vi "Stop Core.vi"(10 "final error code":i32, 11 "Actor in":refnum<class "Actor.lvclass">) -> (3 "Actor out":refnum<class "Actor.lvclass">)   [LabVIEW 2017, in "Actor Framework.lvlib" / "Actor.lvclass"]
doc: "(<B>Filename</B>: Actor Framework.lvlib:Actor.lvclass:Stop Core.vi)\n\nDefines what the actor does before it stops. Use the <B>final error code</B> input to determine whether the actor shut down in response to an error.\n\nBy default, this method does nothing. A descendant class may override it to define behavior, such as shutting down any processes the actor initiated in its override of the Actor Core method."
uses:
  <vilib>/ActorFramework/Actor/Actor.lvclass
  <vilib>/ActorFramework/Actor/Actor.lvclass/Actor.ctl
  <vilib>/ActorFramework/Message Enqueuer/Message Enqueuer.lvclass
  <vilib>/ActorFramework/Stop Msg/Stop Msg.lvclass/Stop Msg.ctl
  <vilib>/ActorFramework/Message Enqueuer/Message Enqueuer.lvclass/Message Enqueuer.ctl
  <vilib>/ActorFramework/Stop Msg/Send Emergency Stop.vi
  <vilib>/ActorFramework/Stop Msg/Send Normal Stop.vi
  <vilib>/ActorFramework/Message Enqueuer/Enqueue Critical.vi
  <vilib>/ActorFramework/Message Enqueuer/Enqueue.vi
  <vilib>/ActorFramework/Stop Msg/Stop Msg.lvclass
  e:/builds/penguin/labview/branches/2017/dev/dist/vi.lib/ActorFramework/Message/Message.lvclass
  <vilib>/ActorFramework/Message Priority Queue/Priority Enqueue.vi
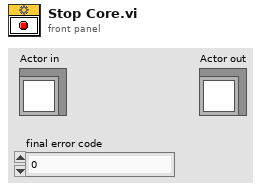
[diagram p1: front panel]
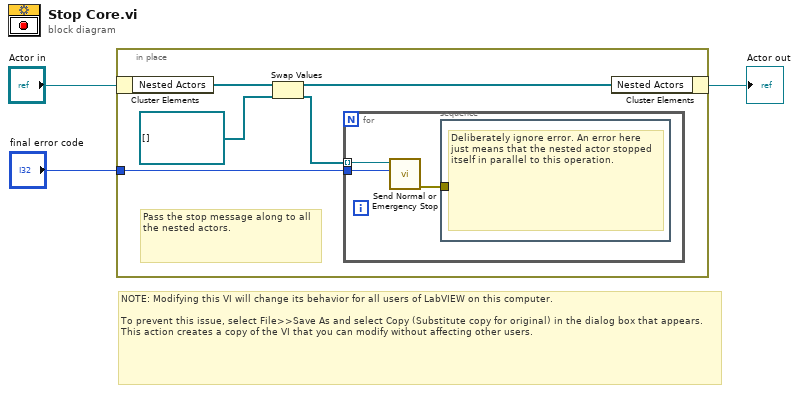
[diagram p0: block diagram]
diagram:
  # "NOTE: Modifying this VI will change its behavior for all users of LabVIEW on this computer.\n\nTo prevent this issue, select File>>Save As and select Copy (Substitute copy for original) in the dialog box that appears. This action creates a copy of the VI that you can modify without affecting other users."
  n1 = in-place {
    in-place-border: "final error code" -> [w4]
    # "Pass the stop message along to all the nested actors."
    n2 = in-place-cluster #1("Actor in") -> ("Nested Actors"=w8:refnum<class "Message Enqueuer.lvclass">[])
    n3 = Swap Values(12:w8, 14:refnum<class "Message Enqueuer.lvclass">[] [] ("Nested Actors")) -> (1:w6:refnum<class "Message Enqueuer.lvclass">[], 3:w5:refnum<class "Message Enqueuer.lvclass">[])  [unwired: 1 in]
    n4 = for {
      tunnel: w5 -> [w11] mode=indexing
      tunnel: w4 -> [w10]
      n5 = call <vilib>:"Send Normal or Emergency Stop.vi"("final error code"=w10, "Message Enqueuer"=w11) -> ("error out"=w9:errorcluster)  [unwired: 9 in]
      n6 = stacked-sequence {
        tunnel: w9 -> [_]
        frame #0 {
          # "Deliberately ignore error. An error here just means that the nested actor stopped itself in parallel to this operation."
        }
      }
    }
    n7 = in-place-cluster #1("Nested Actors"=w6) -> (→"Actor out":refnum<class "Actor.lvclass">)
  }
